vi "曲线判定demo.vi"() -> ()   [LabVIEW 2020]
panel:
  out "添加的数组":string[][](array[string])
  in  "表格控件":string[][](table)
  out "曲线判定条件":T1={"终点位移"=-5.0, "终点误差"=5.0, "判定范围"=[["-5", "-9", "9"], ["6", "-9", "9"]]}
  out "OK？":bool
  in  "Result":string[][](table)
  out "XY图":cluster{dbl[], dbl[]}[](graph)
  in  "文件路径输入控件":path
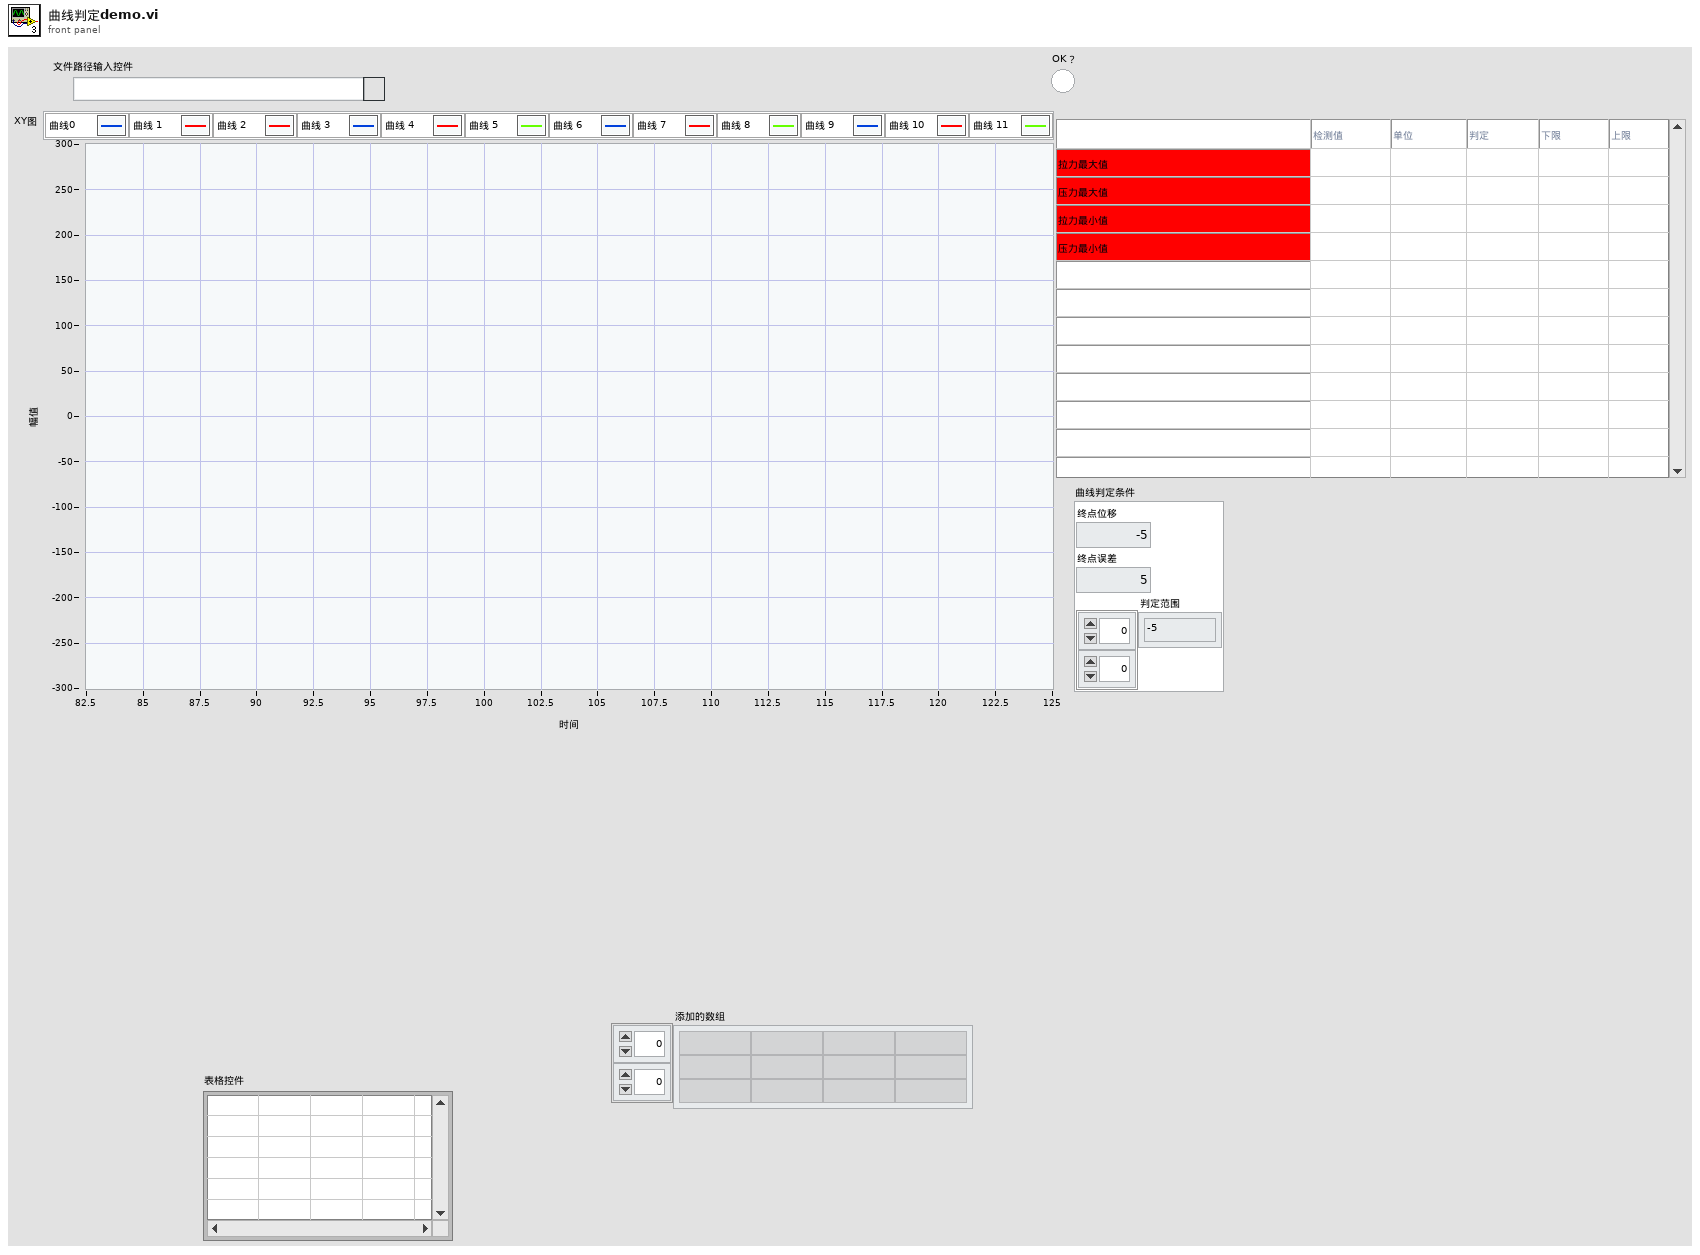
[diagram p1: front panel]
types:
  T1 = cluster{"终点位移":dbl, "终点误差":dbl, "判定范围":string[][]}
  T2 = cluster{"拉力最大值":cluster{"单位":string, "下限":dbl, "上限":dbl}, "压力最大值":cluster{"单位":string, "下限":dbl, "上限":dbl}, "拉力最小值":cluster{"单位":string, "下限":dbl, "上限":dbl}, "压力最小值":cluster{"单位":string, "下限":dbl, "上限":dbl}}
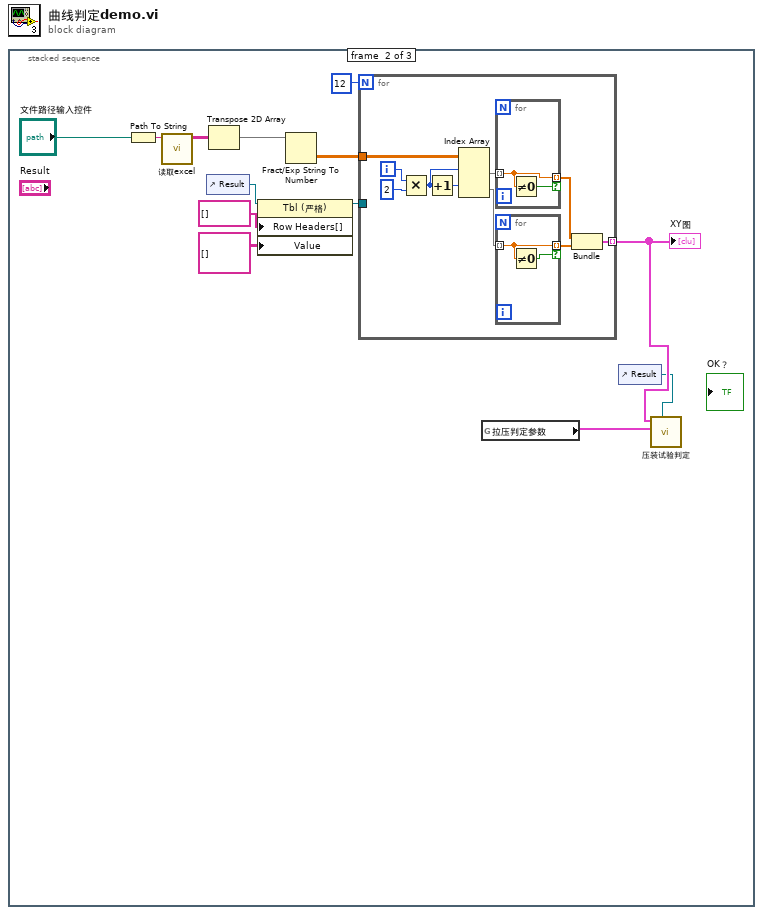
[diagram p0: block diagram]
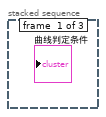
[diagram p2: hidden frame]
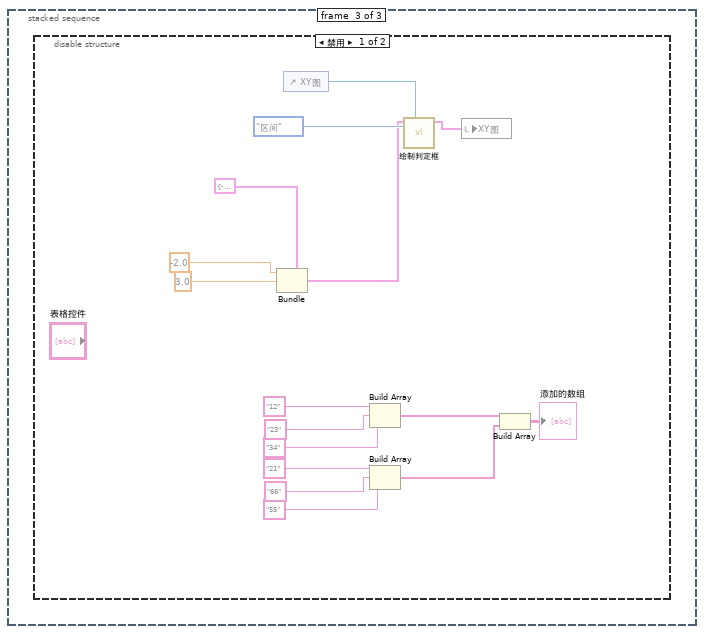
[diagram p3: hidden frame]
diagram:
  n1 = stacked-sequence {
    frame #0 {
    }
    frame #1 {
      n2 = Path To String(path="文件路径输入控件") -> (string=w12:string)
      n3 = call "读取excel.vi"("Filename"=w12) -> ("数据"=w11:string[][])  [unwired: 10 in]
      n4 = control-ref of="Result"() -> (w5:refnum<vi>)
      n5 = Transpose 2D Array(2D array=w11) -> (transposed array=w10:string[][])
      n6 = property class="Tbl (严格)"(reference=w5, "Row Headers[]"=string[] [] ("行首字符串[]"), "Value"=string[][] [] ("值")) -> (reference out=w4:refnum<vi>)  [unwired: 1 in, 1 out]
      n7 = Fract/Exp String To Number(string=w10) -> (number=w9:dbl[][])  [unwired: 3 in, 1 out]
      n8 = for {
        N: 12 -> [_]
        tunnel: w9 -> [w23]
        tunnel: [w17] -> w3 mode=indexing
        tunnel: w4 -> [_]
        i -> [w21]
        n9 = Multiply(x=w21, y=2) -> (x*y=w16:i32)
        n10 = Increment(x=w16) -> (x+1=w15:i32)
        n11 = Index Array(array=w23, index (row) #1=w16, index (row) #2=w15) -> (element #1=w22:dbl[], element #2=w19:dbl[])  [unwired: 2 in]
        n12 = for {
          tunnel: w22 -> [w26] mode=indexing
          tunnel: [w26] -> w18 mode=indexing if=w27
          n13 = Not Equal To 0?(x=w26) -> (x != 0?=w27:bool)
        }
        n14 = for {
          tunnel: w19 -> [w24] mode=indexing
          tunnel: [w24] -> w14 mode=indexing if=w25
          n15 = Not Equal To 0?(x=w24) -> (x != 0?=w25:bool)
        }
        n16 = Bundle(w18, w14) -> (w17:cluster{dbl[], dbl[]})  [unwired: 1 in]
      }
      "XY图" <- w3
      n17 = global read "判定参数.vi" "拉压判定参数"() -> (w1:T2)
      n18 = control-ref of="Result"() -> (w2:refnum<vi>)
      n19 = call "压装试验判定.vi"("Result"=w2, "判定参数"=w1, "XY曲线"=w3) -> ()  [unwired: 7 in, 2 out]
    }
    frame #2 {
      n20 = disable-structure shown="禁用" {
        frame Disabled {
          n21 = Bundle(cluster=T1 {"终点位移"=-5.0, "终点误差"=5.0, "判定范围"=[["-5", "-9", "9"], ["6", "-9", "9"]]} ("曲线判定条件"), "终点位移"=-2.0, "终点误差"=3.0 ("终点位移")) -> (w37:T1)  [unwired: 1 in]
          n22 = control-ref of="XY图"() -> (w43:refnum<vi>)
          n23 = Build Array("12", "23", "34") -> (w33:string[])
          n24 = Build Array("21", "66", "55") -> (w29:string[])
          n25 = call "绘制判定框.vi"("曲线引用"=w43, "判定框类型"=enum16{"区间", "终点"}."区间", "曲线判定条件"=w37) -> ("判定框"=w42:cluster{"横坐标":dbl[], "纵坐标":dbl[]}[])  [unwired: 7 in, 1 out]
          n26 = local write "XY图"(w42) -> ()
          n27 = Build Array(w33, w29) -> (→"添加的数组":string[][])
        }
        frame Enabled {
        }
      }
    }
  }
